vi "cold_cathode_control.vi"(10 "press task in":refnum<k21>, 11 "Cold Cathode Gauge Channel":tag="Dev3/ai6") -> (2 "press task out":refnum<k21>, 3 "Cold Cathode Gauge Pressure":dbl)   [LabVIEW 2014]
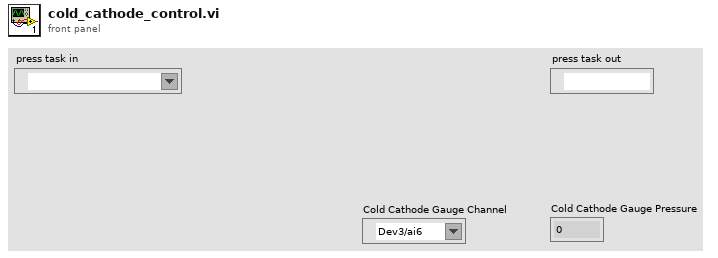
[diagram p1: front panel]
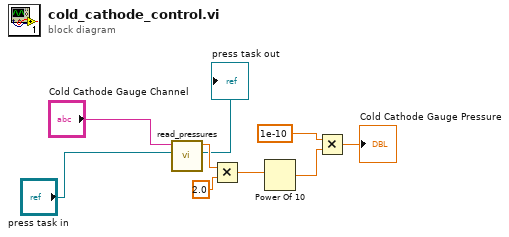
[diagram p0: block diagram]
diagram:
  n1 = call "read_pressures.vi"("press task in"="press task in", "Channel 1"="Cold Cathode Gauge Channel") -> ("press task out"=→"press task out":refnum<k21>, "Ch. 1 value"=w7:dbl)  [unwired: 8 in]
  n2 = Multiply(x=w7, y=2.0) -> (x*y=w5:dbl)
  n3 = Power Of 10(x=w5) -> (10^x=w8:dbl)
  n4 = Multiply(x=1e-10, y=w8) -> (x*y=→"Cold Cathode Gauge Pressure":dbl)
